vi "ASM.Shutdown.vi"(8 "error in (no error)":errorcluster, 11 "ActorStateMachine in":refnum<class "ActorStateMachine.lvclass">) -> (0 "error out":errorcluster, 3 "ActorStateMachine out":refnum<class "ActorStateMachine.lvclass">)   [LabVIEW 2021, in "ActorStateMachine.lvlib" / "ActorStateMachine.lvclass"]
uses:
  ActorStateMachine.lvclass
  _ASM.State.ctl
  ActorStateMachine.lvclass/ActorStateMachine.ctl
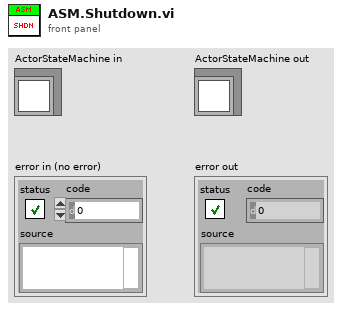
[diagram p1: front panel]
types:
  T1 = typedef "ActorStateMachine.lvlib/ActorStateMachine.lvclass/_ASM.State.ctl" = enum16{"Boom", "Pre-Init", "Init", "Post-Init", "Pre-Reset", "Reset", "Post-Reset", "Pre-Config", "Config", "Post-Config", "Pre-Ready", "Ready", "Post-Ready", "Pre-Running", "Running", "Next", "Post-Running", "Break", "Fail", "Crash", "Shutdown", "Doom"}
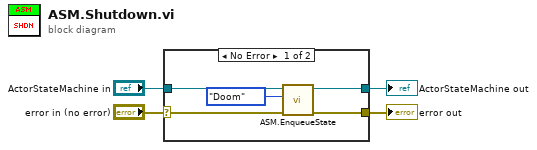
[diagram p0: block diagram]
diagram:
  n1 = case shown="No Error" "error in (no error)" {
    selector: "error in (no error)" -> [w9 w11]
    tunnel: [w8 w11] -> w3
    tunnel: [w7 w10] -> w1
    tunnel: "ActorStateMachine in" -> [w6 w10]
    frame No Error {
      n2 = call "ASM.EnqueueState.vi"("error in (no error)"=w9, "NextState"=_ASM.State."Doom", "ActorStateMachine in"=w6) -> ("error out"=w8:errorcluster, "ActorStateMachine out"=w7:refnum<class "ActorStateMachine.lvclass">)  [unwired: 7 in]
    }
    frame Error {
    }
  }
  "error out" <- w3
  "ActorStateMachine out" <- w1
